vi "Shutdown.vi"(8 "error in":errorcluster, 11 "Chronometer in":refnum<class "Chronometer.lvclass">) -> (0 "error out":errorcluster, 3 "Chronometer out":refnum<class "Chronometer.lvclass">)   [LabVIEW 2023, in "Chronometer.lvlib" / "Chronometer.lvclass"]
uses:
  Chronometer.lvclass
  Chronometer.lvclass/Chronometer.ctl
  Update Record.vi
  Private/Find UUT Record.vi
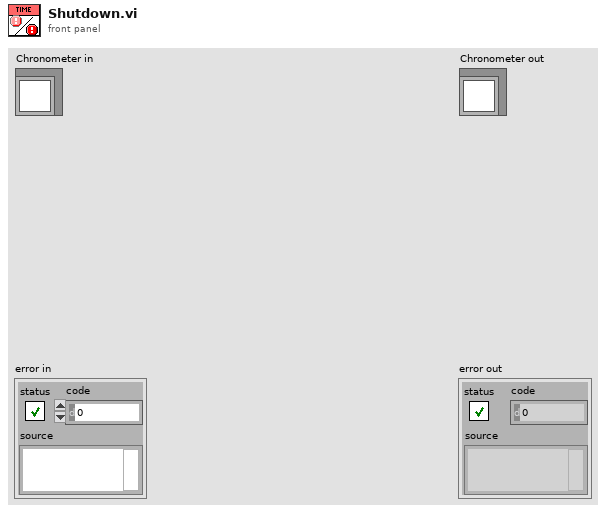
[diagram p1: front panel]
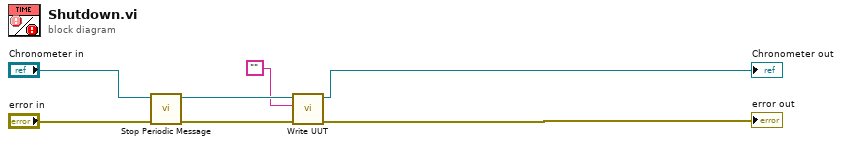
[diagram p0: block diagram]
diagram:
  n1 = call "Stop Periodic Message.vi"("error in"="error in", "Chronometer in"="Chronometer in") -> ("error out"=w4:errorcluster, "Chronometer out"=w5:refnum<class "Chronometer.lvclass">)  [unwired: 8 in]
  n2 = call "Write UUT.vi"("error in"=w4, "UUT"="", "Chronometer in"=w5) -> ("error out"=→"error out":errorcluster, "Chronometer out"=→"Chronometer out":refnum<class "Chronometer.lvclass">)  [unwired: 7 in]
